vi "ConditionalJump.vi"(8 "Current Index":dbl, 9 "Condition":dbl, 11 "Offset":dbl) -> (3 "New Index":dbl)   [LabVIEW 2013]
uses:
  Robot Global Data.vi
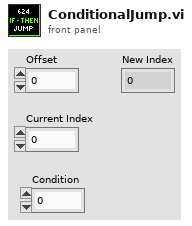
[diagram p1: front panel]
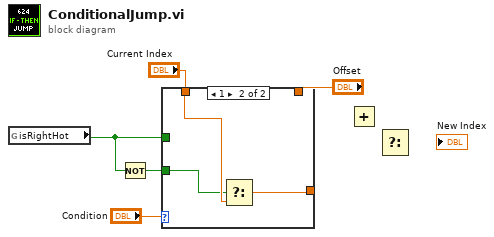
[diagram p0: block diagram]
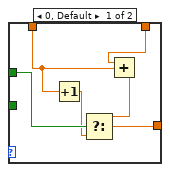
[diagram p2: hidden frame]
diagram:
  n1 = global read "Robot Global Data.vi" "isRightHot"() -> (w2:bool)
  n2 = Not(x=w2) -> (.not. x?=w1:bool)
  n3 = case shown="1" "Condition" {
    tunnel: "Current Index" -> [w8 w14]
    tunnel: "Offset" -> [w11 w15]
    tunnel: [w10 w16] -> w4
    tunnel: w2 -> [w9 _]
    tunnel: w1 -> [_ w13]
    frame 0, Default {
      n4 = Increment(x=w8) -> (x+1=w7:dbl)
      n5 = Add(x=w11, y=w8) -> (x+y=w12:dbl)
      n6 = Select(t=w12, s=w9, f=w7) -> (s? t:f=w10:dbl)
    }
    frame 1 {
      n7 = Select(s=w13, f=w14) -> (t=w17:dbl, s? t:f=w16:dbl)
    }
  }
  n8 = Add() -> ()  [unwired: 2 in, 1 out]
  n9 = Select() -> ()  [unwired: 3 in, 1 out]
